vi "FooterGUI.vi"() -> ()   [LabVIEW 2021, in "Footer.lvclass"]
uses:
  Footer.lvclass
panel:
  out "String":string
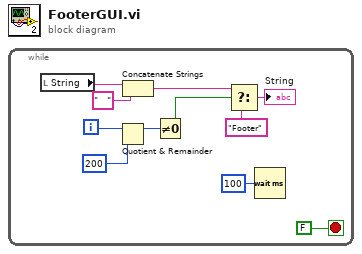
[diagram p0: block diagram]
diagram:
  n1 = while {
    i -> [w11]
    stop <- FALSE stop-if-true
    n2 = local read "String"() -> (w6:string)
    n3 = Quotient & Remainder(x=w11, y=200) -> (x-y*floor(x/y)=w9:i32)  [unwired: 1 out]
    n4 = Concatenate Strings(w6, "   " ("string")) -> (w4:string)
    n5 = Not Equal To 0?(x=w9) -> (x != 0?=w8:bool)
    n6 = Select(t=w4, s=w8, f="Footer") -> (s? t:f=→"String":string)
    n7 = Wait (ms)(milliseconds to wait=u32 100) -> ()  [unwired: 1 out]
  }
